vi "indicator for manual commands.vi"(0 "images":refnum<vi>, 1 "variable":refnum<vi>, 2 "1DArrays":refnum<vi>, 3 "where is the data stored":string[][](array[string]), 4 "config array":string[][](array[string])) -> (5 "appended array":string[][](array[string])=[["localsavingpath", "get,set", "anything", "text"], ["runmode", "get,set", "on,off", "text"], ["save", "get,set", "on,off", "text"], ["trigger", "get,set", "on,off", "text"], ["exposure", "get,set", "NA", "numeric"], ["triggerdelay", "get,set", "NA", "numeric"], ["gain", "get,set", "NA", "numeric"]], 6 "values":string[][](array[string])=[["anything", ""], ["on", "off"], ["on", "off"], ["on", "off"], ["NA", ""], ["NA", ""], ["NA", ""]])   [LabVIEW 2009]
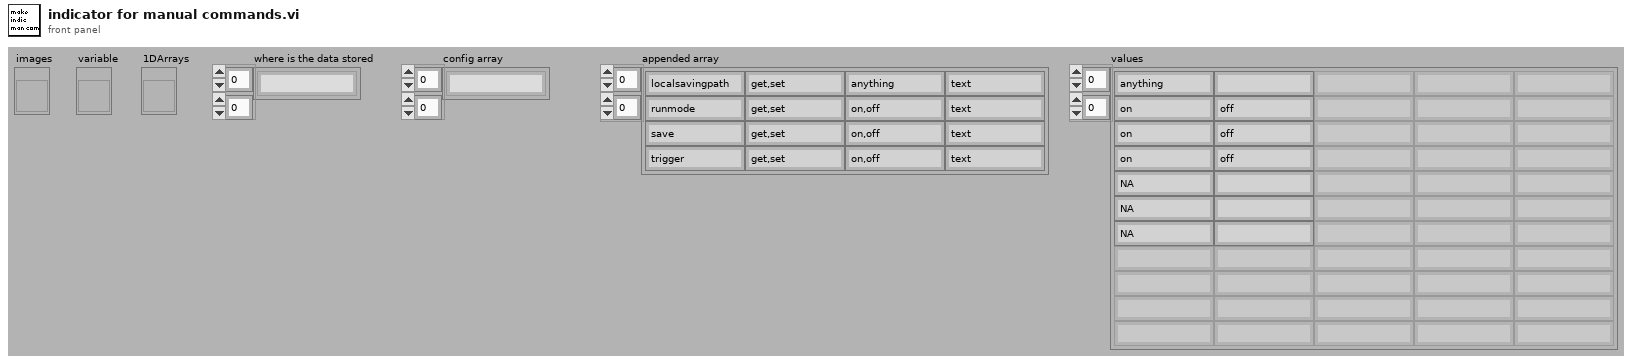
[diagram p1: front panel]
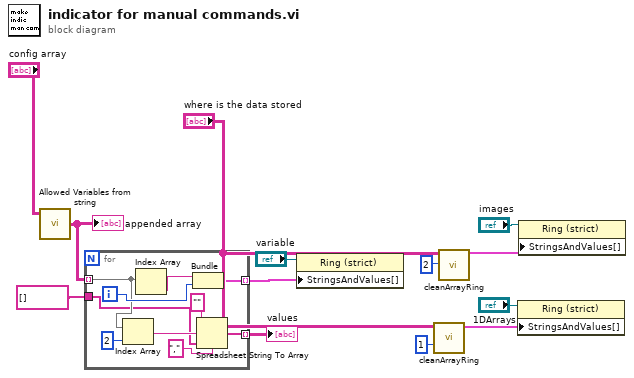
[diagram p0: block diagram]
diagram:
  n1 = call "Allowed Variables from string.vi"("config array 2"="config array") -> ("appended array"=w12:string[][])  [unwired: 4 in]
  "appended array" <- w12
  n2 = for {
    tunnel: w12 -> [w20] mode=indexing
    tunnel: [w22] -> w2 mode=indexing
    tunnel: string[] [] -> [w17]
    tunnel: [w14] -> w4 mode=indexing
    i -> [w21]
    n3 = Index Array(array=w20, index=2) -> (element=w18:string)
    n4 = Index Array(array=w20) -> (element=w23:string)  [unwired: 1 in]
    n5 = Bundle("String"=w23, w21) -> (w22:cluster{"String":string, i32})  [unwired: 1 in]
    n6 = Spreadsheet String To Array(delimiter (Tab)=",", format string="", spreadsheet string=w18, array type (2D Dbl)=w17) -> (array=w14:string[])
  }
  "values" <- w4
  n7 = property class="Ring (strict)"(reference="variable", "StringsAndValues[]"=w2) -> ()  [unwired: 1 in, 2 out]
  n8 = call "cleanArrayRing.vi"("index (row)"=1, "array in"="where is the data stored") -> ("Array out"=w11:cluster{"String":string, i32}[])  [unwired: 9 in]
  n9 = call "cleanArrayRing.vi"("index (row)"=2, "array in"="where is the data stored") -> ("Array out"=w8:cluster{"String":string, i32}[])  [unwired: 9 in]
  n10 = property class="Ring (strict)"(reference="1DArrays", "StringsAndValues[]"=w11) -> ()  [unwired: 1 in, 2 out]
  n11 = property class="Ring (strict)"(reference="images", "StringsAndValues[]"=w8) -> ()  [unwired: 1 in, 2 out]
